vi "Initialize.vi"(8 "error in (no error)":errorcluster, 11 "HoribaCCD in":refnum<class "HoribaCCD.lvclass">) -> (0 "error out":errorcluster, 3 "HoribaCCD out":refnum<class "HoribaCCD.lvclass">)   [LabVIEW 2014, in "DigitizerPlugins.lvlib" / "HoribaCCD.lvclass"]
uses:
  HoribaCCD.lvclass
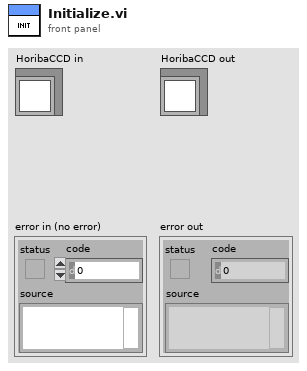
[diagram p1: front panel]
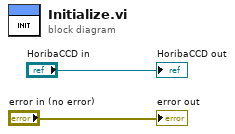
[diagram p0: block diagram]
diagram:
  "error out" <- "error in (no error)"
  "HoribaCCD out" <- "HoribaCCD in"
